vi "_TEST Tests.vi"(4 "error in (no error)":errorcluster) -> (0 "error out":errorcluster)   [LabVIEW 2011]
uses:
  Test Record.ctl
  Test Table Fields.ctl
panel:
  out "Test":T1
  out "Tests":T1[](array[typedef])
  in  "Sort by Field (Name)":T2
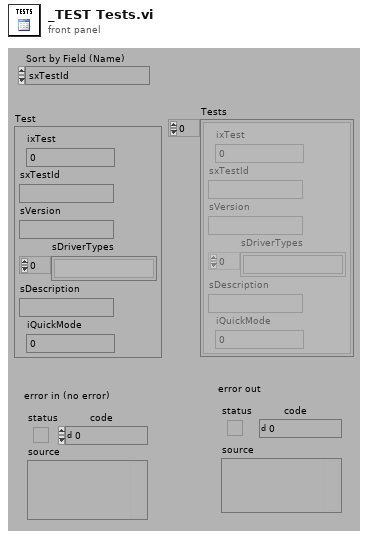
[diagram p1: front panel]
types:
  T1 = typedef "Test Record.ctl" = cluster{"ixTest":i32, "sxTestId":string, "sVersion":string, "sDriverTypes":string[], "sDescription":string, "iQuickMode":i32}
  T2 = typedef "Test Table Fields.ctl" = enum32{"sxTestId", "sVersion", "sDriverTypes", "sDescription", "sQuickMode", "ixTest"}
  T3 = typedef "Connection Refnum.ctl" = cluster{"Environment Handle":i32, "Connection Handle":i32}
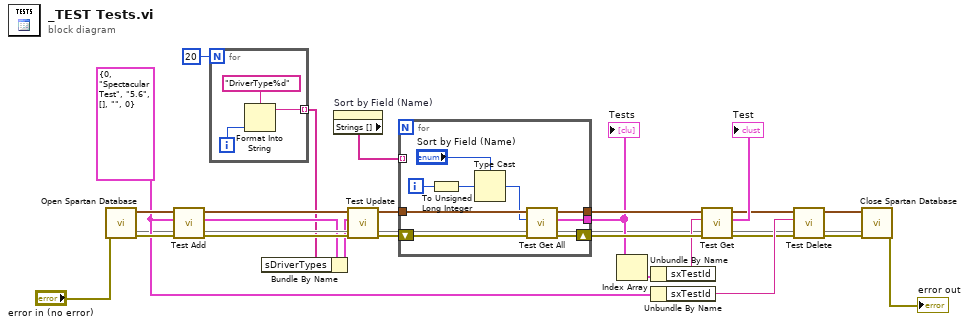
[diagram p0: block diagram]
diagram:
  w16 = T1 {"ixTest"=0, "sxTestId"="Spectacular Test", "sVersion"="5.6", "sDriverTypes"=[], "sDescription"="", "iQuickMode"=0} ("Test Record")
  n1 = call "Open Spartan Database.vi"("error in (no error)"="error in (no error)") -> ("error out"=w26:errorcluster, "Connection Refnum"=w25:T3, 4:w11)  [unwired: 1 in, 7 out]
  n2 = call "Test Add.vi"("error in (no error)"=w26, "Test Record"=w16, "Connection Refnum"=w25) -> ("error out"=w6:errorcluster, "New Test Record"=w4:T1, "Connection Refnum"=w8:T3)  [unwired: 6 out]
  n3 = for {
    N: 20 -> [_]
    tunnel: [w27] -> w2 mode=indexing
    i -> [w28]
    n4 = Format Into String(format string="DriverType%d", w28) -> (resulting string=w27:string)  [unwired: 2 in, 1 out]
  }
  n5 = Bundle By Name(cluster=w4, "sDriverTypes"=w2) -> (w3:T1)
  n6 = property on="Sort by Field (Name)" class="Enum (strict)"() -> ("Strings []"=w24:string[])  [unwired: 2 in, 2 out]
  n7 = call "Test Update.vi"("error in (no error)"=w6, "Test Record"=w3, "Connection Refnum"=w8) -> ("error out"=w5:errorcluster, "Connection Refnum"=w7:T3)  [unwired: 7 out]
  n8 = for {
    shift-right: [w32] -> w22
    shift-left: w5 -> [w33]
    tunnel: w7 -> [w38]
    tunnel: w24 -> [_] mode=indexing
    tunnel: [w31] -> w23
    tunnel: [w30] -> w21
    i -> [w36]
    n9 = To Unsigned Long Integer(number=w36) -> (unsigned 32bit integer=w35:u32)
    n10 = Type Cast(type="Sort by Field (Name)", x=w35) -> (*(type *) &x=w34:T2)
    n11 = call "Test Get All.vi"("error in (no error)"=w33, "Sort by (sxTestId)"=w34, "Connection Refnum"=w38) -> ("error out"=w32:errorcluster, "Test Records"=w30:T1[], "Connection Refnum"=w31:T3)  [unwired: 1 in, 5 out]
  }
  "Tests" <- w21
  n12 = Index Array(array=w21) -> (element=w20:T1)  [unwired: 1 in]
  n13 = Unbundle By Name(w20) -> ("sxTestId"=w19:string)
  n14 = Unbundle By Name(w16) -> ("sxTestId"=w15:string)
  n15 = call "Test Get.vi"("error in (no error)"=w22, "Test_ID"=w19, "Connection Refnum"=w23) -> ("error out"=w14:errorcluster, "Test Record"=→"Test":T1, "Connection Refnum"=w17:T3)  [unwired: 6 out]
  n16 = call "Test Delete.vi"("error in (no error)"=w14, "sxTestId (\"\")"=w15, "Connection Refnum"=w17) -> ("error out"=w12:errorcluster, "Connection Refnum"=w13:T3)  [unwired: 7 out]
  n17 = call "Close Spartan Database.vi"("Force Close? (f)"=w11, "error in (no error)"=w12, "Connection Refnum"=w13) -> ("error out"=→"error out":errorcluster)  [unwired: 1 in, 7 out]
